vi "COMMAND ROM FILE.vi"() -> ()   [LabVIEW 2020]
panel:
  in  "write buffer":string
  out "error out":errorcluster
  out "read buffer":string
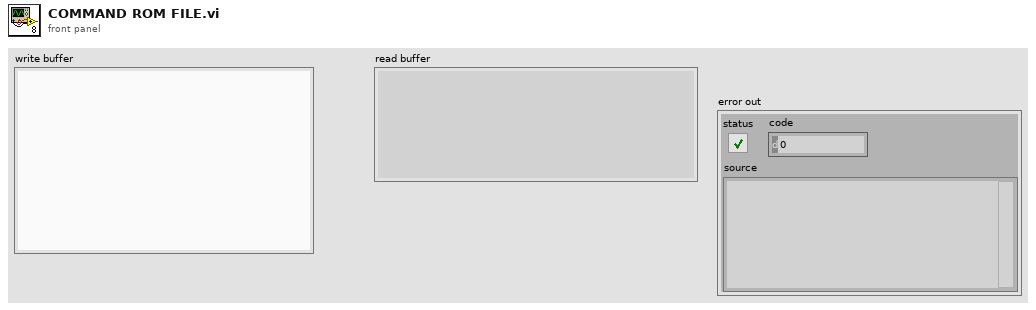
[diagram p1: front panel]
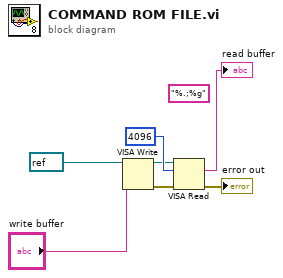
[diagram p0: block diagram]
diagram:
  (unwired) "%.;%g" ("format string")
  n1 = VISA Write(VISA resource name=refnum<visa-resource-name> "USB0::0x0957::0x8E18::MY51140695::INSTR", write buffer="write buffer") -> (VISA resource name out=w6:refnum<visa-resource-name>, error out=w5:errorcluster)  [unwired: 1 in, 1 out]
  n2 = VISA Read(VISA resource name=w6, byte count=u32 4096, error in (no error)=w5) -> (read buffer=→"read buffer":string, error out=→"error out":errorcluster)  [unwired: 2 out]
